vi "Object detection mode FGV.vi"(8 "error in (no error)":errorcluster, 10 "Mode":T1, 11 "Init/R/W State":T2) -> (0 "error out":errorcluster, 3 "Object to detect":T1)   [LabVIEW 2018]
uses:
  Box FGV/Box Colour FGV States.ctl
  Object Detection SubVI/Object Detection SubVI v2 object detection mode.ctl
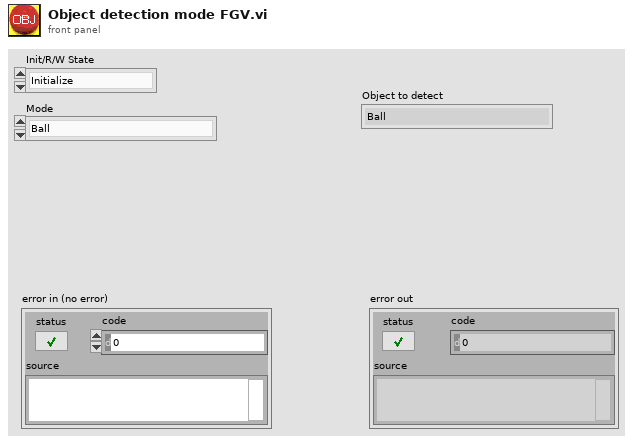
[diagram p1: front panel]
types:
  T1 = typedef "Object Detection SubVI v2 object detection mode.ctl" = enum16{"Ball", "Soap", "Gel", "Pipe", "None"}
  T2 = typedef "Box Colour FGV States.ctl" = enum16{"Initialize", "Read", "Write"}
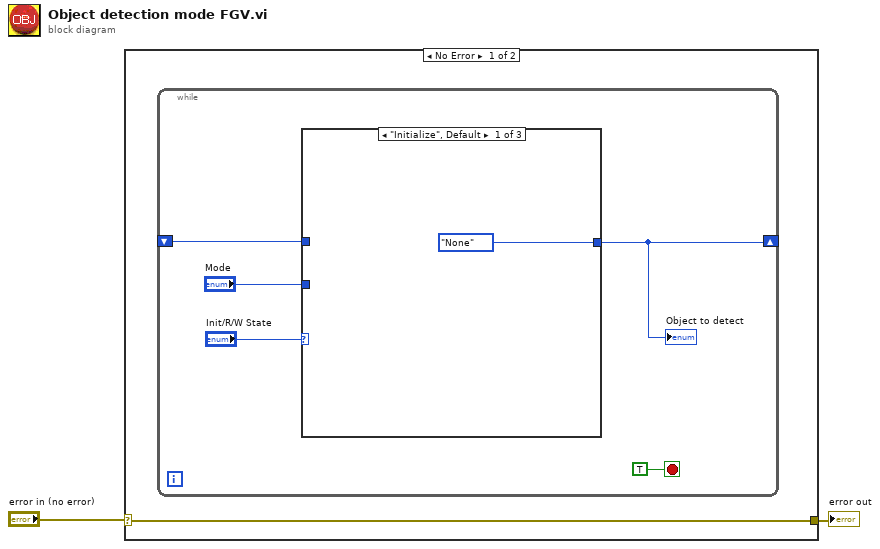
[diagram p0: block diagram]
diagram:
  n1 = case shown="No Error" "error in (no error)" {
    selector: "error in (no error)" -> [w3 w12]
    tunnel: [w3 w12] -> w1
    frame No Error {
      n2 = while {
        shift-right: [w4] -> _
        shift-left: _ -> [w6]
        stop <- TRUE stop-if-true
        n3 = case shown="\"Initialize\", Default" "Init/R/W State" {
          tunnel: [Object_Detection_SubVI_v2_object_detection_mode."None" ("Mode") w10 w11] -> w4
          tunnel: w6 -> [_ w10 _]
          tunnel: "Mode" -> [_ _ w11]
          frame "Initialize", Default {
          }
          frame "Read" {
          }
          frame "Write" {
          }
        }
        "Object to detect" <- w4
      }
    }
    frame Error {
    }
  }
  "error out" <- w1
